vi "checkBackupFiles.vi"(0 "reference in":refnum<class "excelFile.lvclass">, 2 "backup_path":path, 5 "error in (no error)":errorcluster) -> (14 "reference out":refnum<class "excelFile.lvclass">, 16 "backup_path":path, 19 "error out":errorcluster)   [LabVIEW 2016, in "excelFile.lvclass"]
uses:
  excelFile.lvclass
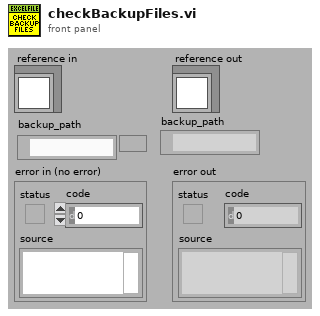
[diagram p1: front panel]
types:
  T1 = typedef "excelFile.lvclass/ObjectAttributesRef.ctl" = refnum<data-value>
  T2 = typedef "excelFile.lvclass/ObjectAttributes.ctl" = cluster{"MyAttribute":dbl, "path":string, "Refnum Excel":cluster{"Excel._Application":refnum<k7>, "Workbooks":refnum<k7>, "Open":refnum<k7>}, "data":string[][][], "save":bool, "fileType":T3, "rowsColor":u32[], "python_ref":refnum<class "python.lvclass">, "items_rows":i32[], "excel_range":i32[][], "TSR":cluster{"number":string, "TSR_path":path, "service_path":path, "email_to":string}, "excel_already_opened?":bool, "file_already_opened?":bool, "excel_protected_opened?":bool, "Refnum Cluster Worksheets":cluster{"Excel._Application":refnum<k7>, "Workbooks":refnum<k7>, "Open":refnum<k7>, "Worksheets":refnum<k7>, "Excel._Worksheet":refnum<k7>}, "#_rows":i32}
  T3 = typedef "excelFile.lvclass/fileType.ctl" = enum16{"devices", "items", "partsTracking", "TSR"}
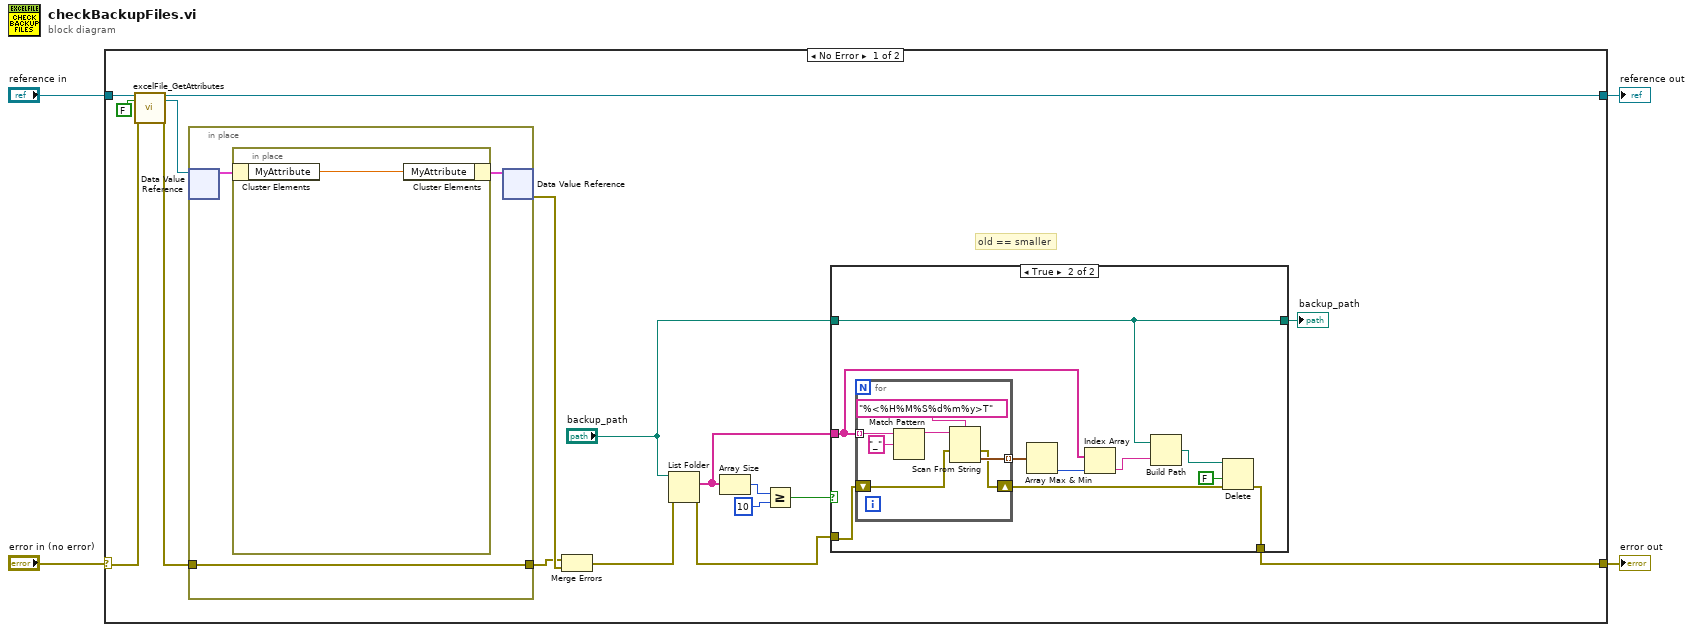
[diagram p0: block diagram]
diagram:
  n1 = case shown="No Error" "error in (no error)" {
    selector: "error in (no error)" -> [w17 w46]
    tunnel: [w6 w46] -> w3
    tunnel: [w15 w45] -> w1
    tunnel: "reference in" -> [w19 w45]
    frame No Error {
      # "old == smaller"
      n2 = call "excelFile_GetAttributes.vi"("reference in"=w19, "return data? (T)"=FALSE, "error in (no error)"=w17) -> ("reference out"=w15:refnum<class "excelFile.lvclass">, "attributes ref"=w14:T1, "error out"=w16:errorcluster)  [unwired: 13 in, 1 out]
      n3 = in-place {
        in-place-border: w16 -> [w41]
        in-place-border: [w41] -> w20
        n4 = in-place-dvr #1(w14) -> (w42:T2)  [unwired: 1 out]
        n5 = in-place {
          n6 = in-place-cluster #2(w42) -> ("MyAttribute"=w44:dbl)
          n7 = in-place-cluster #2("MyAttribute"=w44) -> (w43:T2)
        }
        n8 = in-place-dvr #1(w43) -> (w21:errorcluster)  [unwired: 1 out]
      }
      n9 = Merge Errors(w20, w21) -> (w13:errorcluster)
      n10 = List Folder(path="backup_path", error in=w13) -> (filenames=w9:string[], error out=w7:errorcluster)  [unwired: 2 in, 2 out]
      n11 = Array Size(array=w9) -> (size(s)=w12:i32)
      n12 = Greater Or Equal?(x=w12, y=10) -> (x >= y?=w10:bool)
      n13 = case shown="True" w10 {
        tunnel: w9 -> [_ w31]
        tunnel: "backup_path" -> [w22 w24]
        tunnel: w7 -> [w23 w28]
        tunnel: [w23 w25] -> w6
        tunnel: [w22 w24] -> w5
        frame False {
        }
        frame True {
          n14 = for {
            tunnel: w31 -> [w40] mode=indexing
            tunnel: [w36] -> w33 mode=indexing
            shift-right: [w34] -> w27
            shift-left: w28 -> [w35]
            n15 = Match Pattern(string=w40, regular expression="_") -> (before substring=w37:string)  [unwired: 1 in, 3 out]
            n16 = Scan From String(format string="%<%H%M%S%d%m%y>T", input string=w37, error in=w35) -> (error out=w34:errorcluster, output 1=w36:timestamp)  [unwired: 2 in, 2 out]
          }
          n17 = Array Max & Min(array=w33) -> (min index (indices)=w32:i32)  [unwired: 3 out]
          n18 = Index Array(array=w31, index=w32) -> (element=w30:string)
          n19 = Build Path(base path=w24, name or relative path=w30) -> (appended path=w29:path)
          n20 = Delete(path (use dialog)=w29, confirm (F)=FALSE, error in=w27) -> (error out=w25:errorcluster)  [unwired: 2 in, 2 out]
        }
      }
      "backup_path" <- w5
    }
    frame Error {
    }
  }
  "error out" <- w3
  "reference out" <- w1
